vi "Configure DVM Setting.vi"(8 "error in (no error)":errorcluster, 10 "DVM Setting":T1={"DVM Channel"=1, "Enable DVM Analysis"=FALSE, "Auto Range "=FALSE, "DVM Type"=0} {"DVM Type" items=["Root-mean-square, without DC", "DC Value", "Root-mean-square", "Frequency Counter"]; "DVM Channel" items=["Channel 1"=1, "Channel 2"=2, "Channel 3"=3, "Channel 4"=4]}, 11 "Abstract in":refnum<class "Abstract.lvclass">) -> (0 "error out":errorcluster, 3 "Abstract out":refnum<class "Abstract.lvclass">)   [LabVIEW 2021, in "Oscilloscope.lvlib" / "Abstract.lvclass"]
uses:
  Abstract.lvclass
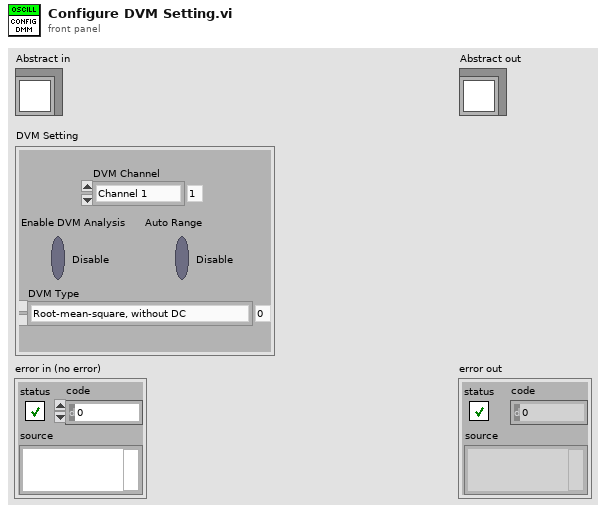
[diagram p1: front panel]
types:
  T1 = cluster{"DVM Channel":i32, "Enable DVM Analysis":bool, "Auto Range ":bool, "DVM Type":i32}
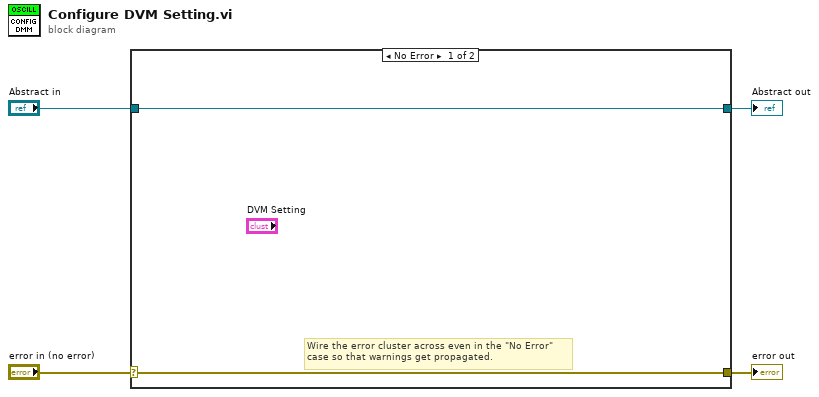
[diagram p0: block diagram]
diagram:
  n1 = case shown="No Error" "error in (no error)" {
    selector: "error in (no error)" -> [w5 w8]
    tunnel: [w5 w8] -> w3
    tunnel: [w6 w7] -> w1
    tunnel: "Abstract in" -> [w6 w7]
    frame No Error {
      # "Wire the error cluster across even in the \"No Error\"\ncase so that warnings get propagated."
    }
    frame Error {
    }
  }
  "error out" <- w3
  "Abstract out" <- w1
